vi "benchmark-memory-tl.vi"() -> ()   [LabVIEW 2020]
uses:
  <vilib>/Platform/TimedLoop/XDataNode/timing_clust.ctl
  <vilib>/Platform/TimedLoop/XDataNode/nitl_modes.ctl
  <vilib>/Platform/TimedLoop/XDataNode/wakeup.ctl
  <vilib>/numeric/Random Number (Range) DBL.vi
  <vilib>/platform/TimedLoop/XDataNode/XDataNode.xnode
  <vilib>/Platform/TimedLoop/XDataNode/XDNodeRunTimeDep.lvlib
panel:
  in  "Period (ms)":i64
  out "processed":i32
  out "wfmg":dbl[][](graph)
  in  "iterations":i32=1000000
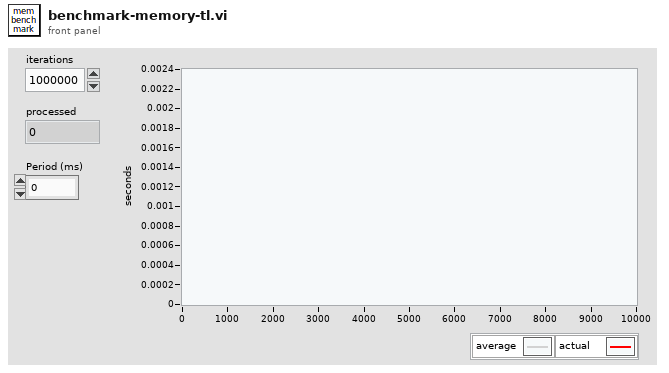
[diagram p1: front panel]
types:
  T1 = typedef "XDNodeRunTimeDep.lvlib/timing_clust.ctl" = cluster{"Expected End [f-1]":u64, "Actual End [f-1]":u64, "Finished Late? [f-1]":bool, "Expected End [i-1]":u64, "Actual End [i-1]":u64, "Finished Late? [i-1]":bool, "Expected Start [i]":u64, "Actual Start [i]":u64, "Expected Start [f]":u64, "Actual Start [f]":u64, "Source Name":string, "Structure Name":string, "Period":i64, "Deadline":i64, "Offset":i64, "Start":i64, "Priority":i32, "Timeout":i32, "Mode":T2, "Wakeup Reason":T3, "Error":errorcluster, "Source Type":string, "Secondary Source Type":string, "Global End Time":u64, "Global Start Time":u64, "Frame Duration":u64, "Iteration Duration":u64, "Assigned CPU":i32, "I/O Scan Engine Mode":u32}
  T2 = typedef "XDNodeRunTimeDep.lvlib/nitl_modes.ctl" = enum32{"No Change", "Process missed periods, maintain original phase", "Discard missed periods, maintain original phase", "Process missed periods, ignore original phase", "Discard missed periods, ignore original phase"}
  T3 = typedef "XDNodeRunTimeDep.lvlib/wakeup.ctl" = enum32{"Normal", "Aborted", "Asynchronous wakeup", "Timing source error", "Timed loop error", "Timeout"}
  T4 = typedef "metadata.ctl" = cluster{"worker ID":u32, "min (s)":dbl, "max (s)":dbl, "mean (s)":dbl, "duration (s)":dbl}
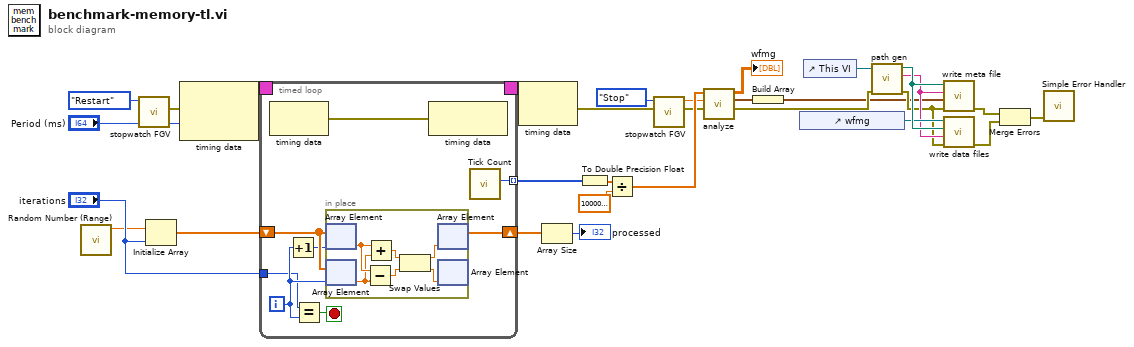
[diagram p0: block diagram]
diagram:
  n1 = call-poly <vilib>:"Random Number (Range).vi"() -> ("number"=w29:dbl)  [unwired: 11 in]
  n2 = call "stopwatch FGV.vi"("state"=enum16{"Restart", "Stop"}."Restart") -> ("error out"=w3:errorcluster)  [unwired: 9 in, 1 out]
  n3 = Initialize Array(w29, "iterations") -> (w28:dbl[])
  n4 = node-c288(w3, "Period (ms)") -> (w8:T1)
  n5 = timed-loop {
    shift-right: [w38] -> w14
    shift-left: w28 -> [w37]
    tunnel: [w35] -> w6 mode=indexing
    timing: w8 -> [_]
    timing-out: [_] -> w7
    tunnel: "iterations" -> [w33]
    i -> [w34]
    stop <- w31 stop-if-true
    n6 = node-c288() -> (w32:errorcluster)  [unwired: 1 in]
    n7 = Increment(x=w34) -> (x+1=w36:i32)
    n8 = Equal?(x=w33, y=w34) -> (x = y?=w31:bool)
    n9 = in-place {
      n10 = in-place-array #1(w37, w36) -> (w46:dbl)
      n11 = in-place-array #2(w37, w34) -> (w45:dbl)
      n12 = Subtract(x=w46, y=w45) -> (x-y=w47:dbl)
      n13 = Add(x=w46, y=w45) -> (x+y=w44:dbl)
      n14 = Swap Values(12:w44, 14:w47) -> (1:w49:dbl, 3:w48:dbl)  [unwired: 1 in]
      n15 = in-place-array #1(w49) -> (w38:dbl[])  [unwired: 1 out]
      n16 = in-place-array #2(w48) -> ()  [unwired: 2 out]
    }
    n17 = node-c288(w32) -> ()  [unwired: 1 out]
    n18 = call "Tick Count"() -> ("Tick Count(uSec)"=w35:u32)
  }
  n19 = node-c288(w7) -> (w2:errorcluster)
  n20 = Array Size(array=w14) -> (size(s)=→"processed":i32)
  n21 = To Double Precision Float(number=w6) -> (double precision float=w5:dbl[])
  n22 = Divide(x=w5, y=1000000.0) -> (x/y=w17:dbl[])
  n23 = call "stopwatch FGV.vi"("error in"=w2, "state"=enum16{"Restart", "Stop"}."Stop") -> ("error out"=w15:errorcluster, "duration (s)"=w16:dbl)  [unwired: 8 in]
  n24 = call "analyze.vi"("error in"=w15, "duration (s)"=w16, "relative seconds"=w17) -> ("error out"=w12:errorcluster, "metadata"=w10:T4, "data"=→"wfmg":dbl[][])  [unwired: 6 in]
  n25 = Build Array(w10) -> (w9:T4[])
  n26 = control-ref of="wfmg"() -> (w23:refnum<vi>)
  n27 = control-ref of="This VI"() -> (w20:refnum<vi>)
  n28 = call "path gen.vi"("error in"=w12, "Calling VI"=w20) -> ("error out"=w11:errorcluster, "basename"=w22:string, "output folder"=w26:path)  [unwired: 7 in]
  n29 = call "write meta file.vi"("error in"=w11, "metadata"=w9, "file basename"=w22, "output folder"=w26) -> ("error out"=w24:errorcluster)  [unwired: 7 in]
  n30 = call "write data files.vi"("error in"=w11, "file basename"=w22, "output folder"=w26, "WaveformGraph in"=w23) -> ("error out"=w25:errorcluster)  [unwired: 7 in]
  n31 = Merge Errors(w24, w25) -> (w27:errorcluster)
  n32 = call <vilib>:"Simple Error Handler.vi"("error in (no error)"=w27) -> ()  [unwired: 4 in, 5 out]
